vi "Assert Pass.vi"(8 "error in (no error)":errorcluster, 9 "Comparator":refnum<class "Comparator.lvclass">, 10 "Mock":refnum<class "Responsive Mock.lvclass">, 11 "Tolerant Numeric Comparator Test In":refnum<class "Tolerant Numeric Comparator Test.lvclass">) -> (0 "error out":errorcluster, 3 "Tolerant Numeric Comparator Test Out":refnum<class "Tolerant Numeric Comparator Test.lvclass">)   [LabVIEW 2020, in "Tolerant Numeric Comparator Test.lvclass"]
uses:
  Tolerant Numeric Comparator Test.lvclass
  source/Framework/Comparator/Comparator.lvclass
  C:/Program Files (x86)/National Instruments/LabVIEW 2020/vi.lib/Astemes/LUnit/Test Case.lvclass
  source/Framework/Responsive Mock/Responsive Mock.lvclass
  <vilib>/Astemes/LUnit/Test Case.lvclass/Test Case.ctl
  <vilib>/Astemes/LUnit/Append Fail Result.vi
  <vilib>/Astemes/LUnit/Append Pass Result.vi
  <vilib>/Astemes/LUnit/Test Case.lvclass
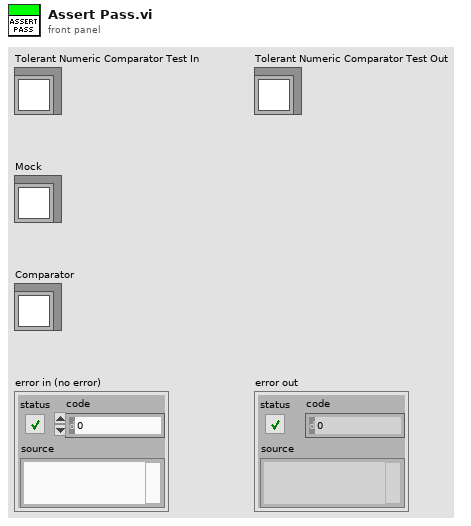
[diagram p1: front panel]
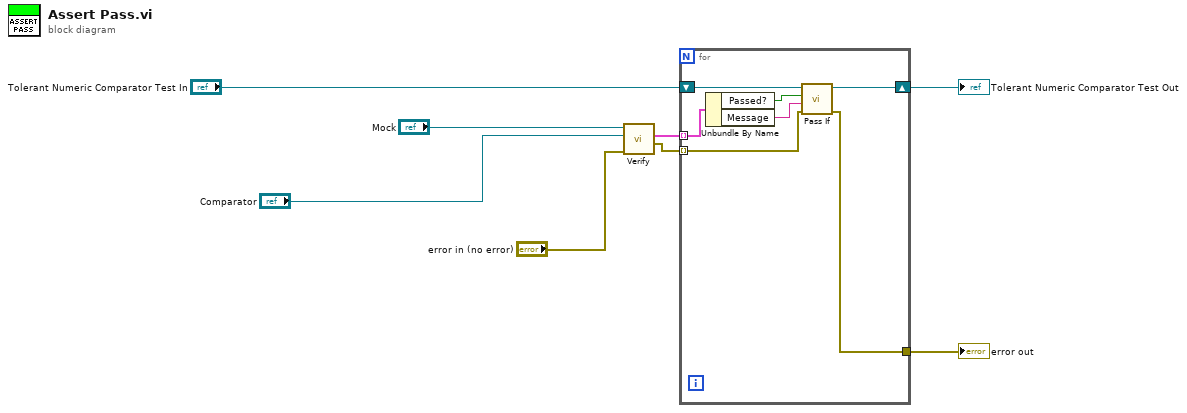
[diagram p0: block diagram]
diagram:
  n1 = call "Verify.vi"("error in (no error)"="error in (no error)", "Comparator"="Comparator", "Mock In"="Mock") -> ("Errors"=w4:errorcluster[], "Results"=w5:cluster{"Passed?":bool, "Message":string}[])  [unwired: 6 in, 1 out]
  n2 = for {
    tunnel: [w14] -> w2
    tunnel: w4 -> [w13] mode=indexing
    tunnel: w5 -> [w11] mode=indexing
    shift-right: [w15] -> w1
    shift-left: "Tolerant Numeric Comparator Test In" -> [w12]
    n3 = Unbundle By Name(w11) -> ("Passed?"=w10:bool, "Message"=w9:string)
    n4 = call <vilib>:"Pass If.vi"("error in (no error)"=w13, "Message"=w9, "Pass?"=w10, "LUnit Test Case In"=w12) -> ("error out"=w14:errorcluster, "LUnit Test Case Out"=w15:refnum<class "Tolerant Numeric Comparator Test.lvclass">)  [unwired: 6 in]
  }
  "error out" <- w2
  "Tolerant Numeric Comparator Test Out" <- w1
